vi "chestdrain.vi"() -> ()   [LabVIEW 2013]
uses:
  <vilib>/Instr/_visa.llb/VISA Configure Serial Port (Instr).vi
panel:
  out "Waveform Chart 4":cluster{"y":dbl, "z":dbl}(graph)
  out "Waveform Chart 3":cluster{i16, i16}(graph)
  out "y":dbl
  out "z":dbl
  in  "d":dbl
  out "d2":dbl
  out "d1":dbl
  out "bot":dbl
  out "top":dbl format="%01.0f"
  out "Waveform Chart 2":cluster{dbl, dbl}(graph)
  in  "escape char":u8=27 format="%x"
  out "read buffer":string
  out "unsigned byte array":u8[](array[numeric])
  out "Waveform Chart":cluster{i32, i32, i32, i32, i32, i32}(graph)
  in  "VISA resource name":refnum<visa-resource-name>="COM1"
  in  "stop":bool
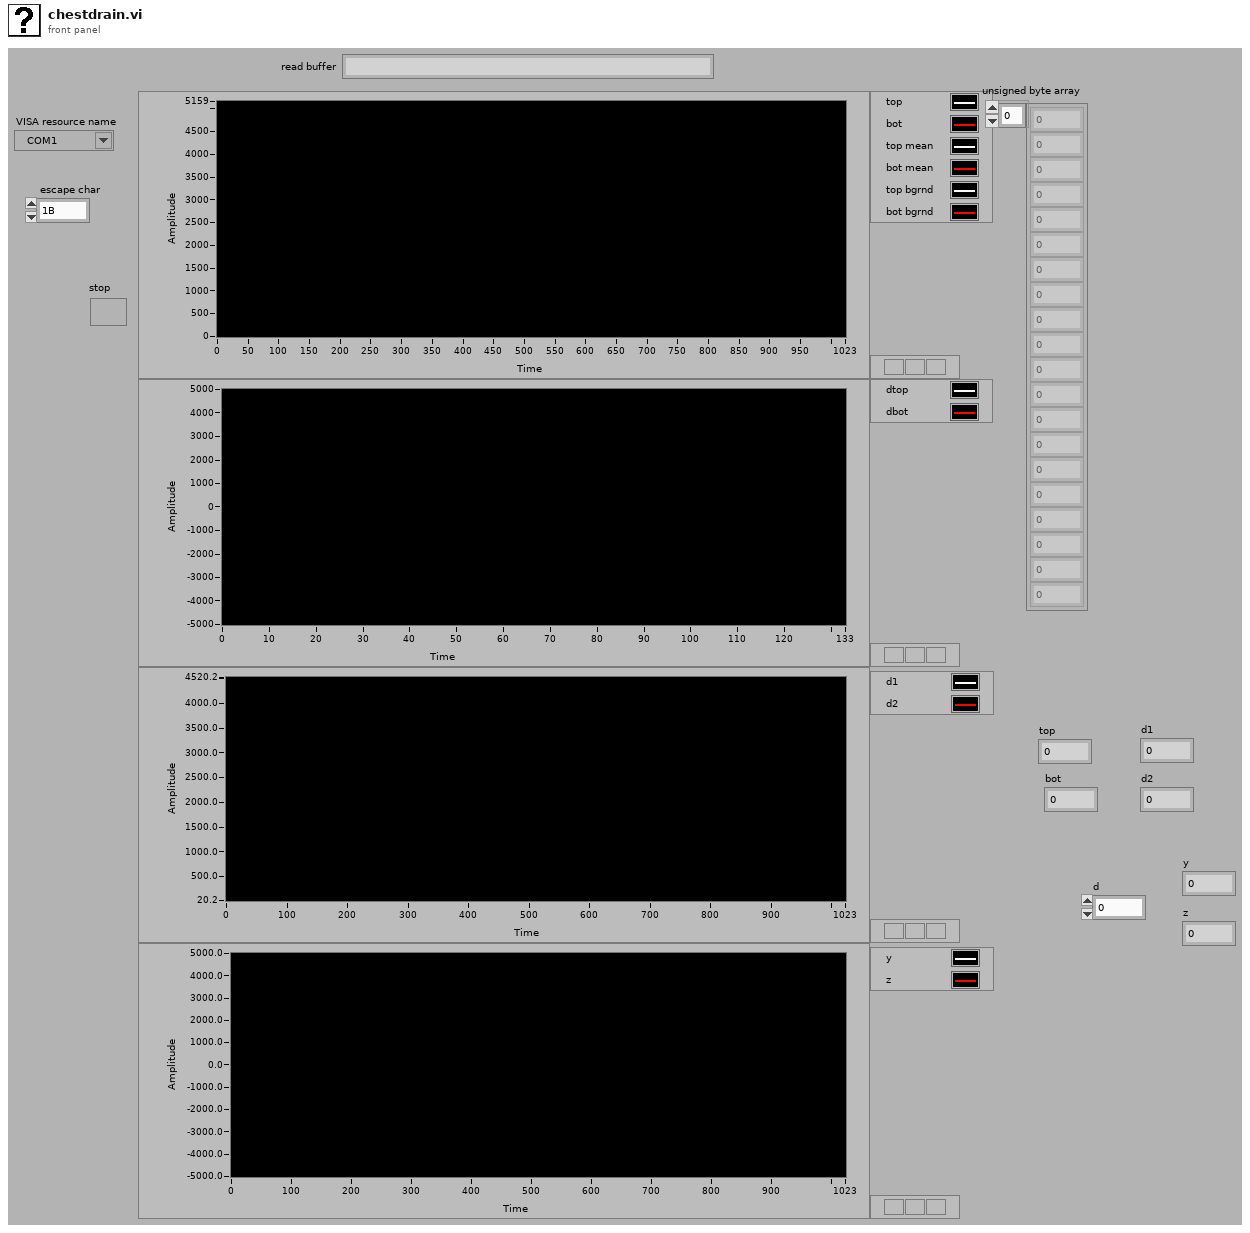
[diagram p1: front panel]
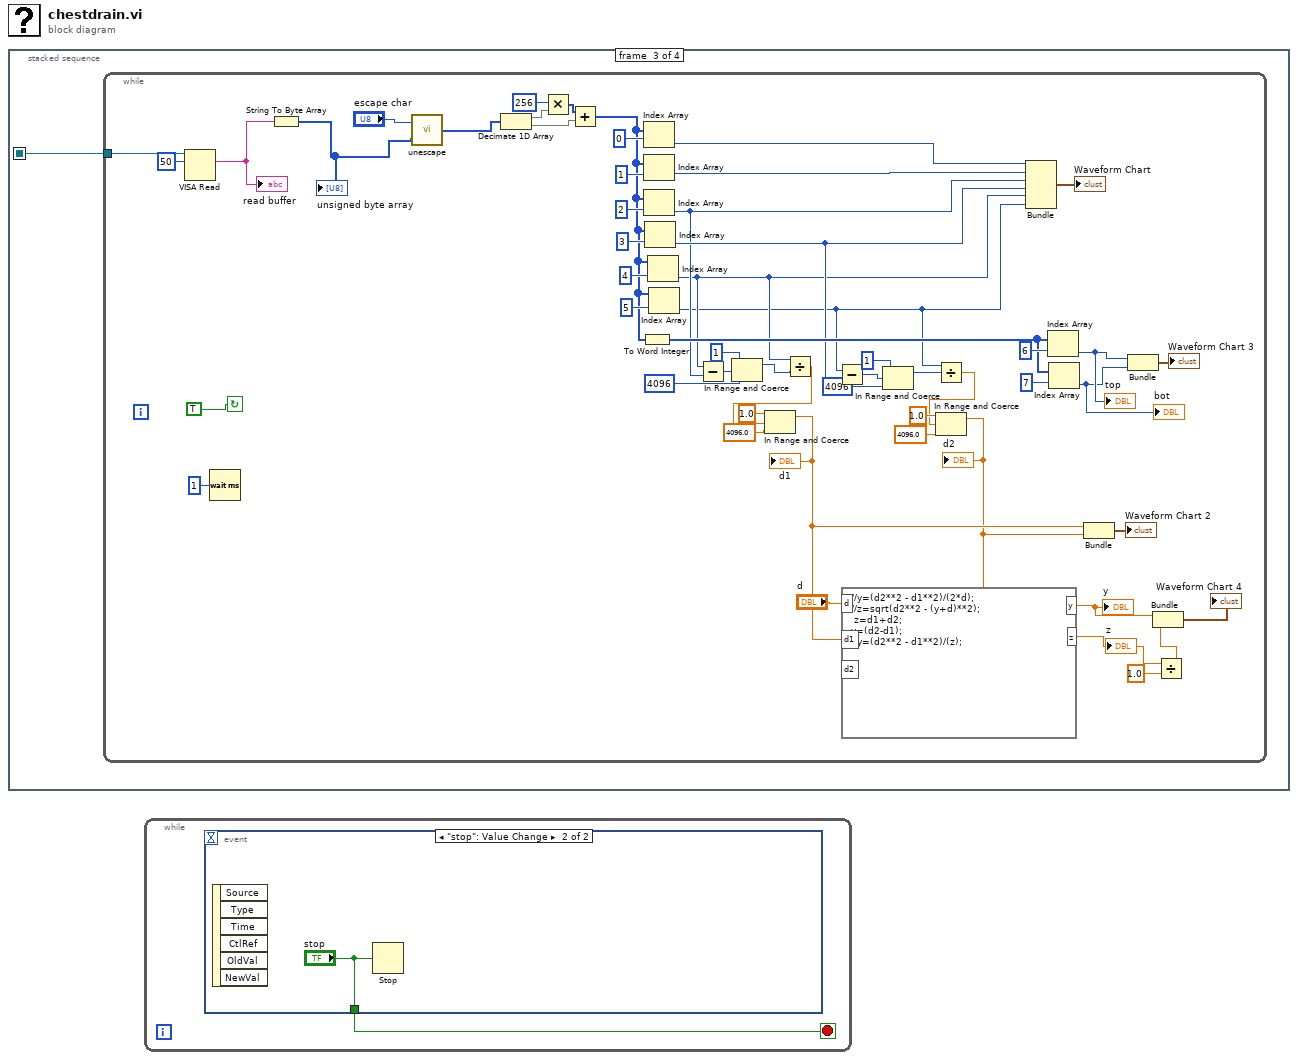
[diagram p0: block diagram]
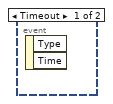
[diagram p2: hidden frame]
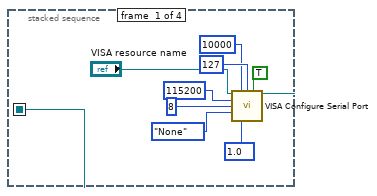
[diagram p3: hidden frame]
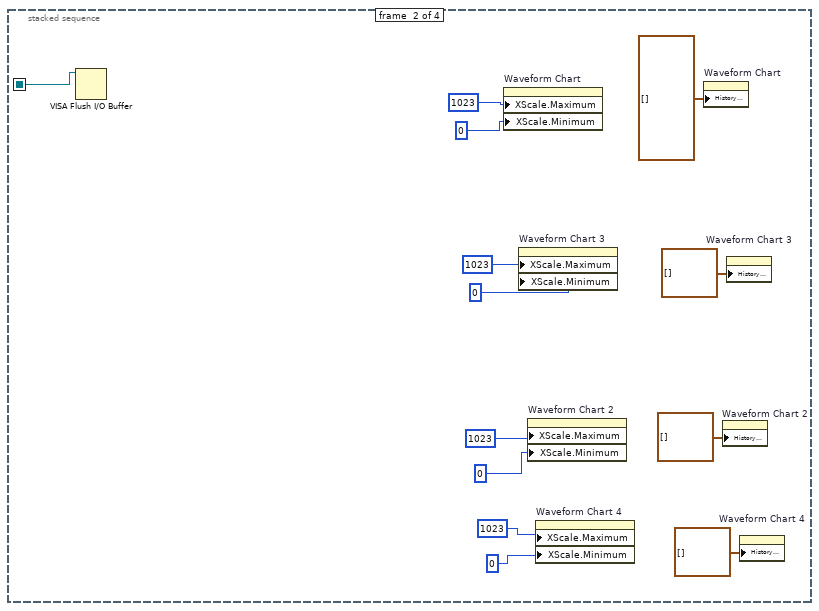
[diagram p4: hidden frame]
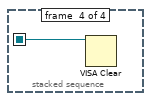
[diagram p5: hidden frame]
diagram:
  n1 = stacked-sequence {
    seq-local: [w5 _ _ _] -> [_ w22 w23 w80]
    frame #0 {
      w7 = u16 10 items=["1.0"=10, "1.5"=15, "2.0"=20] ("stop bits (10: 1 bit)")
      n2 = call-poly "VISA Configure Serial Port"("VISA resource name"="VISA resource name", "timeout (10sec)"=u32 10000, "termination char\n(0xA = '\\n' = LF)"=u8 127 ("termination char\n(0xA = '\\n' = LF)"), "Enable Termination\nChar (T)"=TRUE, "baud rate (9600)"=u32 115200, "data bits (8)"=u16 8, "parity (0:none)"=enum16{"None", "Odd", "Even", "Mark", "Space"}."None", "stop bits (10: 1 bit)"=w7) -> ("VISA resource name out"=w5:refnum<visa-resource-name>)  [unwired: 6 in, 1 out]
    }
    frame #1 {
      n3 = VISA Flush I/O Buffer(VISA resource name=w22) -> ()  [unwired: 2 in, 2 out]
      n4 = property on="Waveform Chart" class="WFChart (strict)"("XScale.Maximum"=1023, "XScale.Minimum"=0) -> ()  [unwired: 2 in, 2 out]
      n5 = property on="Waveform Chart 3" class="WFChart (strict)"("XScale.Maximum"=1023, "XScale.Minimum"=0) -> ()  [unwired: 2 in, 2 out]
      n6 = property on="Waveform Chart 2" class="WFChart (strict)"("XScale.Maximum"=1023, "XScale.Minimum"=0) -> ()  [unwired: 2 in, 2 out]
      n7 = property on="Waveform Chart 4" class="WFChart (strict)"("XScale.Maximum"=1023, "XScale.Minimum"=0) -> ()  [unwired: 2 in, 2 out]
      n8 = property on="Waveform Chart" class="WFChart (strict)"("History Data"=cluster{i32, i32, i32, i32, i32, i32}[] []) -> ()  [unwired: 2 in, 2 out]
      n9 = property on="Waveform Chart 2" class="WFChart (strict)"("History Data"=cluster{dbl, dbl}[] []) -> ()  [unwired: 2 in, 2 out]
      n10 = property on="Waveform Chart 3" class="WFChart (strict)"("History Data"=cluster{i32, i32}[] []) -> ()  [unwired: 2 in, 2 out]
      n11 = property on="Waveform Chart 4" class="WFChart (strict)"("History Data"=cluster{"y":dbl, "z":dbl}[] []) -> ()  [unwired: 2 in, 2 out]
    }
    frame #2 {
      w24 = 0
      n12 = Initialize Array(w24, w24) -> ()  [unwired: 1 out]
      n13 = while {
        tunnel: w23 -> [w70]
        stop <- TRUE continue-if-true
        n14 = VISA Read(VISA resource name=w70, byte count=u32 50) -> (read buffer=w60:string)  [unwired: 1 in, 3 out]
        "read buffer" <- w60
        n15 = Wait (ms)(milliseconds to wait=u32 1) -> ()  [unwired: 1 out]
        n16 = String To Byte Array(string=w60) -> (unsigned byte array=w61:u8[])
        "unsigned byte array" <- w61
        n17 = call "unescape.vi"("byte array in"=w61, "escape character"="escape char") -> ("byte array out"=w67:u8[])
        n18 = Decimate 1D Array(w67) -> (w78:u8[], w76:u8[])
        n19 = Multiply(x=256, y=w78) -> (x*y=w75:i32[])
        n20 = Add(x=w75, y=w76) -> (x+y=w54:i32[])
        n21 = To Word Integer(number=w54) -> (16bit integer=w53:i16[])
        n22 = Index Array(array=w54, index=0) -> (element=w65:i32)
        n23 = Index Array(array=w54, index=1) -> (element=w63:i32)
        n24 = Index Array(array=w54, index=2) -> (element=w49:i32)
        n25 = Index Array(array=w54, index=3) -> (element=w50:i32)
        n26 = Index Array(array=w54, index=4) -> (element=w29:i32)
        n27 = Index Array(array=w54, index=5) -> (element=w28:i32)
        n28 = Subtract(x=w29, y=w49) -> (x-y=w42:i32)
        n29 = In Range and Coerce(upper limit=1, x=w42, lower limit=4096) -> (coerced(x)=w39:i32)  [unwired: 1 out]
        n30 = Divide(x=w29, y=w39) -> (x/y=w48:dbl)
        n31 = In Range and Coerce(upper limit=1.0, x=w48, lower limit=4096.0 ("x")) -> (coerced(x)=w34:dbl)  [unwired: 1 out]
        "d1" <- w34
        n32 = Subtract(x=w28, y=w50) -> (x-y=w36:i32)
        n33 = In Range and Coerce(upper limit=1, x=w36, lower limit=4096) -> (coerced(x)=w35:i32)  [unwired: 1 out]
        n34 = Divide(x=w28, y=w35) -> (x/y=w44:dbl)
        n35 = In Range and Coerce(upper limit=1.0, x=w44, lower limit=4096.0 ("x")) -> (coerced(x)=w33:dbl)  [unwired: 1 out]
        "d2" <- w33
        n36 = formula code="//y=(d2**2 - d1**2)/(2*d);\n//z=sqrt(d2**2 - (y+d)**2);\n z=d1+d2;\ny=(d2-d1);\n//y=(d2**2 - d1**2)/(z);"("d"="d", "d1"=w34, "d2"=w33) -> ("y"=w31:dbl, "z"=w26:dbl)
        "y" <- w31
        "z" <- w26
        n37 = Bundle(w65, w63, w49, w50, w29, w28) -> (→"Waveform Chart":cluster{i32, i32, i32, i32, i32, i32})  [unwired: 1 in]
        n38 = Index Array(array=w53, index=6) -> (element=w52:i16)
        "top" <- w52
        n39 = Index Array(array=w53, index=7) -> (element=w51:i16)
        "bot" <- w51
        n40 = Bundle("upper limit"=w34, "upper limit"=w33) -> (→"Waveform Chart 2":cluster{"upper limit":dbl, "upper limit":dbl})  [unwired: 1 in]
        n41 = Bundle(w52, w51) -> (→"Waveform Chart 3":cluster{i16, i16})  [unwired: 1 in]
        n42 = Divide(x=w26, y=1.0) -> (x/y=w27:dbl)
        n43 = Bundle("y"=w31, w27) -> (→"Waveform Chart 4":cluster{"y":dbl, dbl})  [unwired: 1 in]
      }
    }
    frame #3 {
      n44 = VISA Clear(VISA resource name=w80) -> ()  [unwired: 1 in, 2 out]
    }
  }
  n45 = while {
    stop <- w81 stop-if-true
    n46 = event shown="[1] \"stop\": Value Change" {
      selector: _ -> [_ _]
      dyn-events: _ -> [_ _]
      timeout: _ -> [_ _]
      tunnel: [_ "stop"] -> w81
      event Timeout {
        n47 = event-data() -> ()  [unwired: 1 in, 2 out]
      }
      event "stop": Value Change {
        n48 = event-data() -> ()  [unwired: 1 in, 6 out]
        n49 = Stop(stop? (T)="stop") -> ()
      }
    }
  }
